vi "SVM_Decay.vi"(6 "Hs":dbl[][](array[numeric]), 8 "GapCutOff":i16, 9 "Matrix V":T1, 10 "Matrix S":T1, 11 "Matrix U":T1) -> (1 "G2":dbl[][](array[numeric]), 2 "eigen lamda":dbl[](array[numeric]) min=0.0 max=127.0 format="%.2e", 3 "Eigenvalues":cdb[](array[numeric]), 4 "A(tau)":dbl[](array[numeric]), 5 "Ci":dbl[](array[numeric]))   [LabVIEW 2022 SP3]
uses:
  <vilib>/Analysis/Matrix/Datatypes/RealMatrix.ctl
  <vilib>/Analysis/7linalg.llb/Real Transpose Matrix.vi
  <vilib>/Analysis/7linalg.llb/Real Matrix Square Root.vi
  <vilib>/Analysis/baseanly.llb/Complex A x B.vi
  <vilib>/Analysis/7linalg.llb/Complex Eigenvalues and Vectors.vi
  <vilib>/Analysis/baseanly.llb/Complex Inverse Matrix.vi
  <vilib>/Analysis/7linalg.llb/Create Special Complex Matrix.vi
  <vilib>/Analysis/Matrix/Numeric/Complex/Complex To Cartesian - CM.vi
  <vilib>/Analysis/NI_AALBase.lvlib
  <vilib>/Analysis/NI_AALPro.lvlib
  <vilib>/Analysis/Matrix/NI_Matrix.lvlib
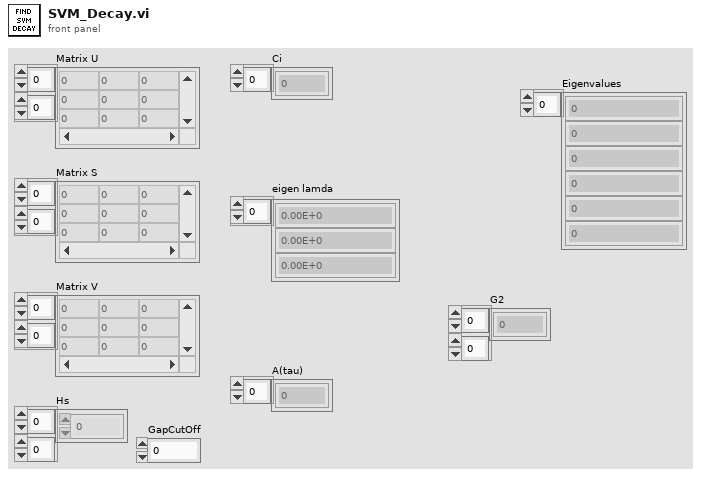
[diagram p1: front panel]
types:
  T1 = typedef "NI_Matrix.lvlib/RealMatrix.ctl" = dbl[][]
  T2 = typedef "NI_Matrix.lvlib/ComplexMatrix.ctl" = cdb[][]
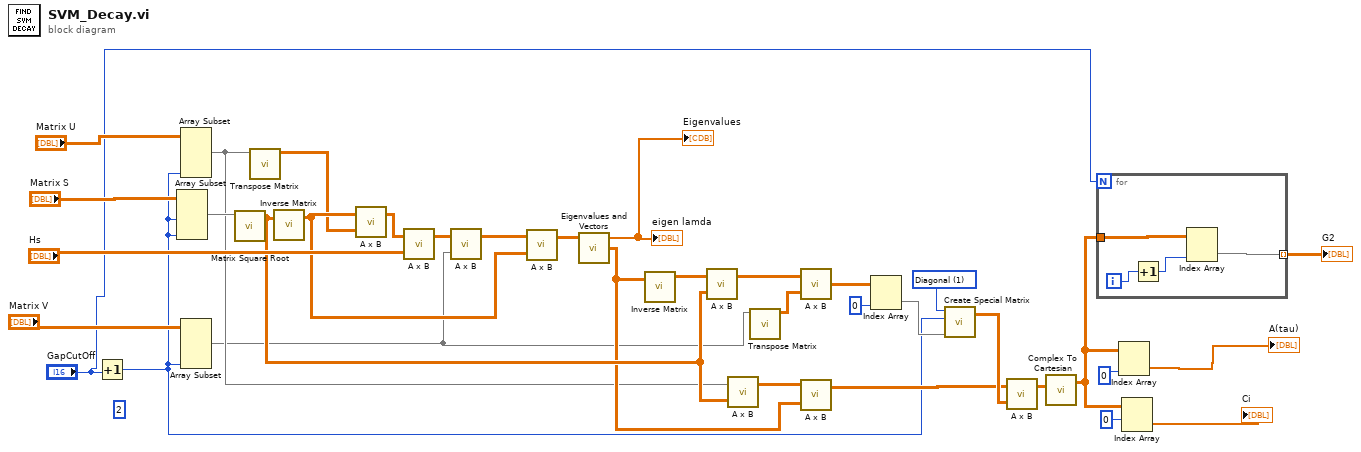
[diagram p0: block diagram]
diagram:
  w17 = 1 items=["Identity", "Diagonal", "Toeplitz", "Vandermonde", "Companion", "Hankel", "Hadamard", "Wilkinson", "Hilbert", "Inverse Hilbert", "Rosser", "Pascal"] ("matrix type")
  (unwired) 2 ("length")
  n1 = Increment(x="GapCutOff") -> (x+1=w2:i16)
  n2 = Array Subset(array="Matrix S", length (row)=w2, length (col)=w2) -> (w28:T1)  [unwired: 2 in]
  n3 = Array Subset(array="Matrix U", length (col)=w2) -> (w15:T1)  [unwired: 3 in]
  n4 = Array Subset(array="Matrix V", length (col)=w2) -> (w11:T1)  [unwired: 3 in]
  n5 = call-poly <vilib>:"Matrix Square Root.vi"("Input Matrix"=w28) -> ("Matrix Square Root"=w30:T2)  [unwired: 1 in, 1 out]
  n6 = call-poly <vilib>:"Transpose Matrix.vi"("Input Matrix"=w15) -> ("Matrix Transpose"=w4:T1)  [unwired: 9 in, 1 out]
  n7 = call-poly <vilib>:"Inverse Matrix.vi"("Input Matrix"=w30) -> ("Inverse Matrix"=w29:T2)  [unwired: 1 in, 1 out]
  n8 = call-poly <vilib>:"A x B.vi"("B"=w4, "A"=w29) -> ("A x B"=w5:T2)  [unwired: 1 out]
  n9 = call-poly <vilib>:"A x B.vi"("B"="Hs", "A"=w5) -> ("A x B"=w6:T2)  [unwired: 1 out]
  n10 = call-poly <vilib>:"A x B.vi"("B"=w11, "A"=w6) -> ("A x B"=w7:T2)  [unwired: 1 out]
  n11 = call-poly <vilib>:"A x B.vi"("B"=w29, "A"=w7) -> ("A x B"=w8:T2)  [unwired: 1 out]
  n12 = call-poly <vilib>:"Eigenvalues and Vectors.vi"("Input Matrix"=w8) -> ("Eigenvectors"=w16:T2, "Eigenvalues"=→"eigen lamda" →"Eigenvalues":cdb[])  [unwired: 2 in, 1 out]
  n13 = call-poly <vilib>:"Inverse Matrix.vi"("Input Matrix"=w16) -> ("Inverse Matrix"=w9:T2)  [unwired: 1 in, 1 out]
  n14 = call-poly <vilib>:"A x B.vi"("B"=w30, "A"=w9) -> ("A x B"=w13:T2)  [unwired: 1 out]
  n15 = call-poly <vilib>:"A x B.vi"("B"=w30, "A"=w15) -> ("A x B"=w14:T2)  [unwired: 1 out]
  n16 = call-poly <vilib>:"Transpose Matrix.vi"("Input Matrix"=w11) -> ("Matrix Transpose"=w12:T1)  [unwired: 9 in, 1 out]
  n17 = call-poly <vilib>:"A x B.vi"("B"=w12, "A"=w13) -> ("A x B"=w18:T2)  [unwired: 1 out]
  n18 = call-poly <vilib>:"A x B.vi"("B"=w16, "A"=w14) -> ("A x B"=w21:T2)  [unwired: 1 out]
  n19 = Index Array(array=w18, index (col)=0 ("disabled index (col)")) -> (element=w20:cdb[])  [unwired: 1 in]
  n20 = call-poly <vilib>:"Create Special Matrix.vi"("matrix type"=w17, "matrix size"=w2, "Input Vector1"=w20) -> ("Special Matrix"=w22:T2)  [unwired: 2 in, 1 out]
  n21 = call-poly <vilib>:"A x B.vi"("B"=w22, "A"=w21) -> ("A x B"=w25:T2)  [unwired: 1 out]
  n22 = call-poly <vilib>:"Complex To Cartesian.vi"("Complex Matrix R + Ii"=w25) -> ("Real Matrix R"=w27:T1)  [unwired: 1 out]
  n23 = for {
    N: "GapCutOff" -> [_]
    tunnel: [w39] -> w32 mode=indexing
    tunnel: w27 -> [w38]
    i -> [w37]
    n24 = Increment(x=w37) -> (x+1=w36:i32)
    n25 = Index Array(array=w38, index (col)=w36) -> (element=w39:dbl[])  [unwired: 1 in]
  }
  "G2" <- w32
  n26 = Index Array(array=w27, index (col)=0 ("disabled index (col)")) -> (element=→"A(tau)":dbl[])  [unwired: 1 in]
  n27 = Index Array(array=w27, index (row)=0) -> (element=→"Ci":dbl[])  [unwired: 1 in]
